vi "parse_EndEffectorState.vi"(4 "error in":errorcluster, 7 "msg in":string) -> (0 "error out":errorcluster, 2 "EndEffectorState":T1, 3 "msg out":string)   [LabVIEW 2010]
uses:
  std_msgs/subs/parse_u32_scalar.vi
  std_msgs/subs/parse_float32_scalar.vi
  std_msgs/subs/parse_time_scalar.vi
  std_msgs/subs/parse_string_array.vi
  std_msgs/subs/parse_u8_array.vi
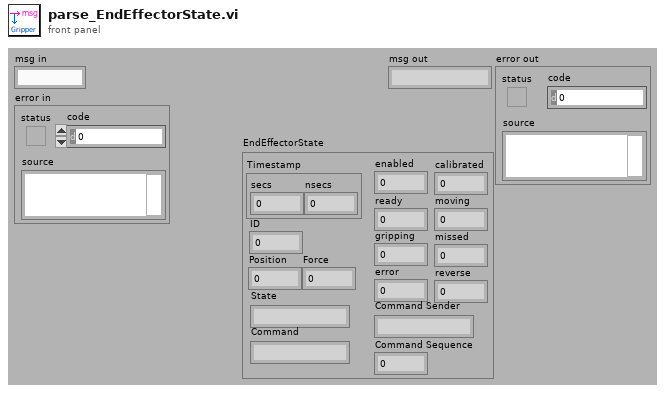
[diagram p1: front panel]
types:
  T1 = cluster{"Timestamp":cluster{"secs":i32, "nsecs":i32}, "ID":u32, "enabled":u8, "calibrated":u8, "ready":u8, "moving":u8, "gripping":u8, "missed":u8, "error":u8, "reverse":u8, "Position":sgl, "Force":sgl, "State":string, "Command":string, "Command Sender":string, "Command Sequence":u32}
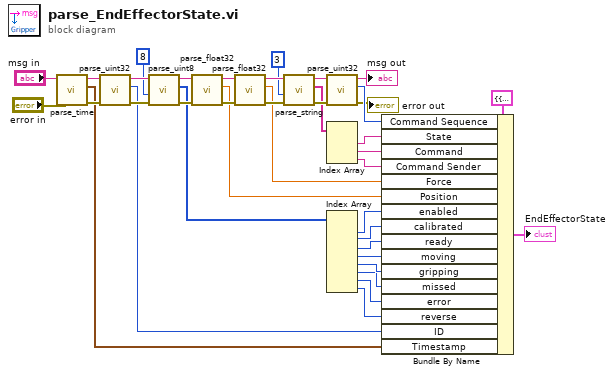
[diagram p0: block diagram]
diagram:
  n1 = call-poly "parse_time.vi"("error in"="error in", "msg in"="msg in") -> ("error out"=w38:errorcluster, "Time"=w4:cluster{"secs":i32, "nsecs":i32}, "msg out"=w37:string)  [unwired: 3 in]
  n2 = call-poly "parse_uint32.vi"("error in"=w38, "msg in"=w37) -> ("error out"=w36:errorcluster, "number"=w5:u32, "msg out"=w35:string)  [unwired: 3 in]
  n3 = call-poly "parse_uint8.vi"("error in"=w36, "Array Size"=8, "msg in"=w35) -> ("error out"=w30:errorcluster, "number"=w21:u8[], "msg out"=w31:string)  [unwired: 2 in]
  n4 = call-poly "parse_float32.vi"("error in"=w30, "msg in"=w31) -> ("error out"=w33:errorcluster, "number"=w14:sgl, "msg out"=w32:string)  [unwired: 3 in]
  n5 = call-poly "parse_float32.vi"("error in"=w33, "msg in"=w32) -> ("error out"=w29:errorcluster, "number"=w15:sgl, "msg out"=w28:string)  [unwired: 3 in]
  n6 = call-poly "parse_string.vi"("error in"=w29, "Array Size"=3, "msg in"=w28) -> ("error out"=w26:errorcluster, "strings"=w19:string[], "msg out"=w25:string)  [unwired: 2 in]
  n7 = call-poly "parse_uint32.vi"("error in"=w26, "msg in"=w25) -> ("error out"=→"error out":errorcluster, "number"=w20:u32, "msg out"=→"msg out":string)  [unwired: 3 in]
  n8 = Index Array(array=w19) -> (element #1=w18:string, element #2=w17:string, element #3=w16:string)  [unwired: 3 in]
  n9 = Index Array(array=w21) -> (element #1=w13:u8, element #2=w12:u8, element #3=w11:u8, element #4=w10:u8, element #5=w9:u8, element #6=w8:u8, element #7=w7:u8, element #8=w6:u8)  [unwired: 8 in]
  n10 = Bundle By Name(cluster=T1 {"Timestamp"={"secs"=0, "nsecs"=0}, "ID"=0, "enabled"=0, "calibrated"=0, "ready"=0, "moving"=0, "gripping"=0, "missed"=0, "error"=0, "reverse"=0, "Position"=0.0, "Force"=0.0, "State"="", "Command"="", "Command Sender"="", "Command Sequence"=0} ("EndEffectorState"), "Command Sequence"=w20, "State"=w18, "Command"=w17, "Command Sender"=w16, "Force"=w15, "Position"=w14, "enabled"=w13, "calibrated"=w12, "ready"=w11, "moving"=w10, "gripping"=w9, "missed"=w8, "error"=w7, "reverse"=w6, "ID"=w5, "Timestamp"=w4) -> (→"EndEffectorState":T1)
